vi "UNIXTimeToString.vi"(10 "dt":u64) -> (2 "DateTime":string)   [LabVIEW 2015]
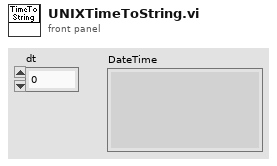
[diagram p1: front panel]
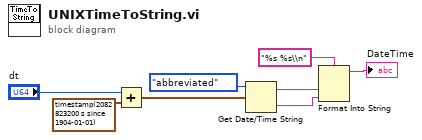
[diagram p0: block diagram]
diagram:
  n1 = Add(x="dt", y=timestamp(2082823200 s since 1904-01-01)) -> (x+y=w7:timestamp)
  n2 = Get Date/Time String(date format (0)=enum16{"short", "long", "abbreviated"}."abbreviated", seconds (now)=w7) -> (date string=w3:string, time string=w2:string)  [unwired: 1 in]
  n3 = Format Into String(format string="%s %s\\n", w3, w2) -> (resulting string=→"DateTime":string)  [unwired: 2 in, 1 out]
